vi "estructura eventos.vi"() -> ()   [LabVIEW 2016]
panel:
  out "Numeric Control":i32
  out "Boolean 2":bool
  in  "Boolean":bool
  in  "Stop Button":bool
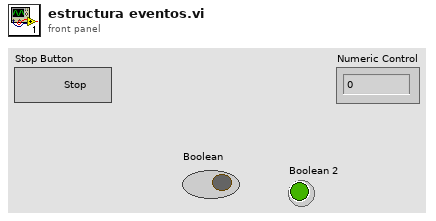
[diagram p1: front panel]
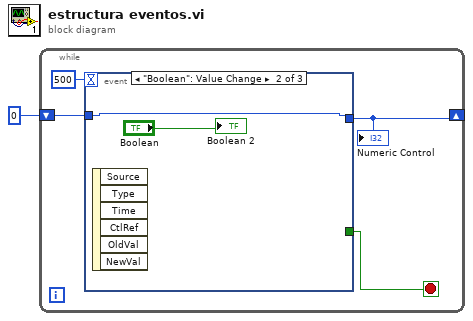
[diagram p0: block diagram]
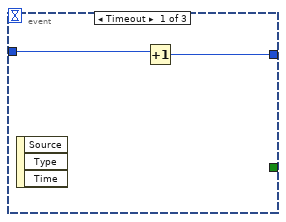
[diagram p2: hidden frame]
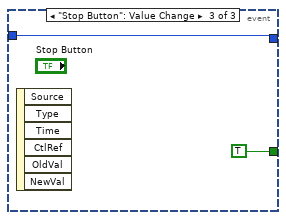
[diagram p3: hidden frame]
diagram:
  n1 = while {
    shift-right: [w3] -> _
    shift-left: 0 -> [w4]
    stop <- w5 stop-if-true
    n2 = event shown="[1] \"Boolean\": Value Change" {
      selector: _ -> [_ _ _]
      dyn-events: _ -> [_ _ _]
      timeout: 500 -> [_ _ _]
      tunnel: [_ _ TRUE] -> w5
      tunnel: w4 -> [w7 w8 w10]
      tunnel: [w6 w8 w10] -> w3
      event Timeout {
        n3 = event-data() -> ()  [unwired: 1 in, 3 out]
        n4 = Increment(x=w7) -> (x+1=w6:i32)
      }
      event "Boolean": Value Change {
        n5 = event-data() -> ()  [unwired: 1 in, 6 out]
        "Boolean 2" <- "Boolean"
      }
      event "Stop Button": Value Change {
        n6 = event-data() -> ()  [unwired: 1 in, 6 out]
      }
    }
    "Numeric Control" <- w3
  }
